vi "TrajectoryConfig_GetConstraints.vi"(11 "inTRAJECTORY_CONFIG":T1 {"End Velocity" format="%20.4f"; "StartVelocity" format="%20.4f"; "Max Acceleration" format="%20.4f"; "MaxVelocity" format="%20.4f"}) -> (3 "Constraints":variant[](array[variant]))   [LabVIEW 2019, in "Trajectory_Library.lvlib"]
doc: "Return the array of Contraints contained in the Trajectory Configuration.\n\nParameters:\n - InTrajectoryConfig - The trajectory configuration data structure\n\nReturns:\n - Constraints -- Array of variants containing the data clusters for trajjectory constraints.\n\n - OutTrajectoryConfig - Modified trajectory configuration data structure"
uses:
  Trajectory_Library.lvlib
  TypeDef/TRAJ_CONFIG.ctl
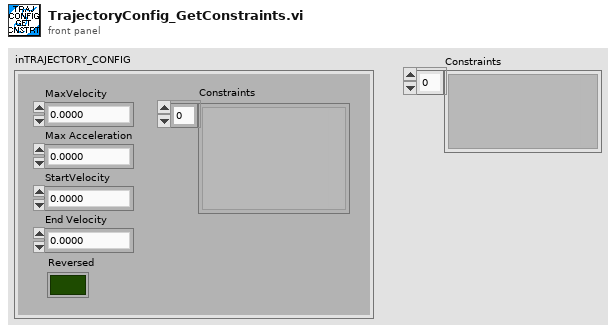
[diagram p1: front panel]
types:
  T1 = typedef "Trajectory_Library.lvlib/TRAJ_CONFIG.ctl" = cluster{"MaxVelocity":dbl, "Max Acceleration":dbl, "StartVelocity":dbl, "End Velocity":dbl, "Reversed":bool, "Constraints":variant[]}
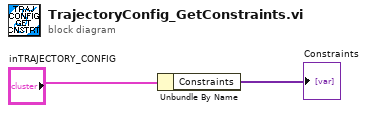
[diagram p0: block diagram]
diagram:
  n1 = Unbundle By Name("inTRAJECTORY_CONFIG") -> ("Constraints"=→"Constraints":variant[])
